vi "Sequence.vi"() -> ()   [LabVIEW 2016]
uses:
  Sequence.Action.ctl
  Sequence.Data.ctl
  Sequence.State.ctl
  Sequence.Step.Status.ctl
  Sequence.Test.BreakReason.ctl
  Sequence.Test.BreakSource.ctl
  Sequence.Test.Status.ctl
  Sequence.Slot.StatusData.ctl
  Sequence.Test.Unload.Status.ctl
  Sequence.Prod.StatusData.ctl
  Sequence.UserActions.ctl
  Sequence.UserData.ctl
  Sequence.MainMode.ctl
  Gui/MainGui.TestOptions.ctl
  Sequence.Code.Sets.ctl
  Sequence.PlateType.ctl
  Logger/Logger.Variant.Sets.ctl
  Station/Station.Changeover.State.vi
  Station/Station.Plate.Properties.ctl
  Sequence.Code.SerialFormat.ctl
  Drivers/V7310/LowLevel/V7310.Job.Sets.ctl
  Sequence.Counters.ctl
  tools/CitTemplate/citTemplate.errData.ctl
  tools/EventLog/EventLog.EventSource.ctl
  tools/Translator/Translator.Message.ctl
  Station/Station.ValvePosition.ctl
  Drivers/FestoCPX/Station/FestoCPX.Station.ProdArmPosition.ctl
  Station/Station.ProductSlot.ctl
  Sequence.SerialsFglb.Action.ctl
  Sequence.UserAction.ctl
  Sequence.Global.vi
  Station/Station.Global.vi
  Drivers/V7310/LowLevel/V7310.Global.vi
panel:
  out "SuckerLastStates":bool[](array[boolean])
  out "Data":T1={"BeginTS"=timestamp(0 s since 1904-01-01), "EndTS"=timestamp(0 s since 1904-01-01), "State"=enum."Init", "Status.Work"=enum."-", "Status.Process"=enum."-", "Status.Home"=enum."-", "Status.Wabco"=enum."-", "Status.Client"=enum."-", "BreakReason"=enum."-", "BreakSource"=enum."-", "DoorLock"=FALSE, "Status.Prod"=[], "UserAction"={"Stop"=FALSE, "Pause"=FALSE, "Next"=FALSE}, "UserData"={"GuiMode"=enum."Process", "Test"={"IgnoreResults"=FALSE, "IgnoreImages"=FALSE, "ServiceMode"=FALSE}, "ContinueOrder"=FALSE}, "Error"={"status"=FALSE, "code"=0, "source"=""}, "Code"={"Ready"=FALSE, "DoubleOrder"=FALSE, "OrderDone"=FALSE, "AllowSingleSlot"=FALSE, "CheckDM"=FALSE, "ThresholdA"=0, "ThresholdB"=0, "Plate"=enum."Wabco", "ImgPath"=path "", "Variant"={"State"=enum."Init", "ImgPath"=path "", "WabcoPlate"="", "WabcoProduct"="", "ClientProduct"="", "ClientPlate"="", "TotalQuantity"=0, "OrderQuantity"=0, "Serial"=0, "Wabco"={"LaserJob"="", "AdditionalTxt"="037", "FactoryCode"="", "RevID"=0, "ForkID"=0, "FailuresLimit"=0, "GlobalCnt"=0, "ScannerProgram"=0, "SerialFormat"=enum."6 dig", "CoordA"={"X"=0.0, "Y"=0.0, "Angle"=0.0}, "CoordB"={"X"=0.0, "Y"=0.0, "Angle"=0.0}, "DMCconfig"=0}, "Client"={"LaserJob"="", "AdditionalTxt"="", "FactoryCode"="037", "RevID"=0, "ForkID"=0, "FailuresLimit"=0, "GlobalCnt"=0, "ScannerProgram"=0, "SerialFormat"=enum."6 dig", "CoordA"={"X"=0.0, "Y"=0.0, "Angle"=0.0}, "CoordB"={"X"=0.0, "Y"=0.0, "Angle"=0.0}, "DMCconfig"=0}}}, "Rotations"=0, "ProdIdx"=0, "ProdDone"=[], "PrintedSerials-Wabco"=[], "PrintedSerials-Client"=[], "Counters-Wabco"={"Expected"=0, "Done"=0, "OK"=0, "NOK"=0, "NOKlimit"=0, "Part"=0, "PartOK"=0}, "Counters-Client"={"Expected"=0, "Done"=0, "OK"=0, "NOK"=0, "NOKlimit"=0, "Part"=0, "PartOK"=0}}
  out "action":T22=enum."--- Sequence ---"
  out "_loop":i32(ring)=4
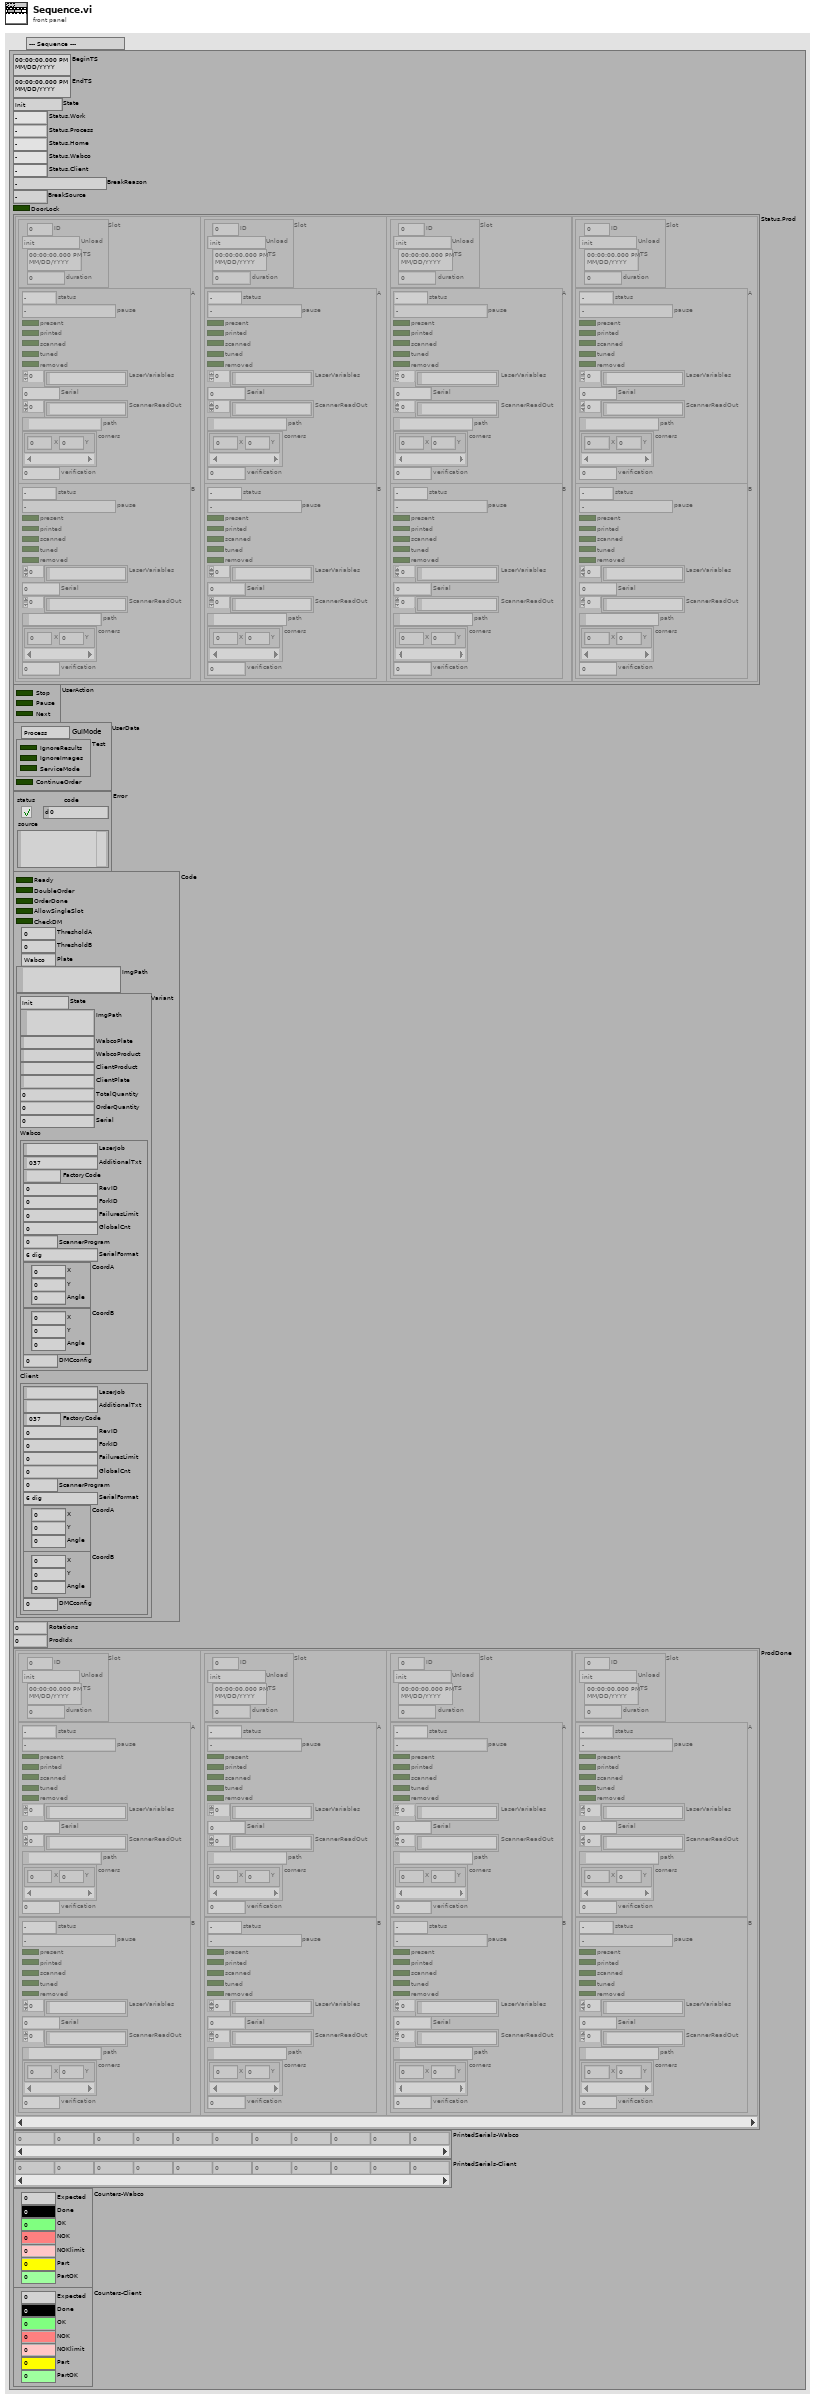
[diagram p1: front panel]
types:
  T1 = typedef "Sequence.Data.ctl" = cluster{"BeginTS":timestamp, "EndTS":timestamp, "State":T2, "Status.Work":T3, "Status.Process":T3, "Status.Home":T3, "Status.Wabco":T3, "Status.Client":T3, "BreakReason":T4, "BreakSource":T5, "DoorLock":bool, "Status.Prod":T6[], "UserAction":T10, "UserData":T11, "Error":errorcluster, "Code":T14, "Rotations":i32, "ProdIdx":i32, "ProdDone":T6[], "PrintedSerials-Wabco":i32[], "PrintedSerials-Client":i32[], "Counters-Wabco":T21, "Counters-Client":T21}
  T2 = typedef "Sequence.State.ctl" = enum16{"Init", "Idle", "Home", "Work", "Run", "Pause"}
  T3 = typedef "Sequence.Step.Status.ctl" = enum16{"-", "Pending", "Running", "Skipped", "Passed", "Failed", "Done", "Error", "Aborted", "Stopped"}
  T4 = typedef "Sequence.Test.BreakReason.ctl" = enum16{"-", "NOK container", "OK container", "Rev empty", "Rev missing", "Rev wrong", "Fork missing", "Fork wrong", "NOK limit", "Unload failure", "Single slot", "Part done", "Err: Prod move work", "Err: Prod move home", "Err: Prod lift work", "Err: Prod lift home", "Err: Prod Arm Work", "Err: Prod Arm NOK", "Err: Prod Arm OK", "Err: Prod NOK suck", "Err: Prod NOK drop", "Err: Prod OK missing", "Err: Prod OK suck", "Err: Prod OK drop"}
  T5 = typedef "Sequence.Test.BreakSource.ctl" = enum16{"-", "A", "B", "A/B"}
  T6 = typedef "Sequence.Test.Status.ctl" = cluster{"Slot":T7, "A":T9, "B":T9}
  T7 = typedef "Sequence.Slot.StatusData.ctl" = cluster{"ID":i32, "Unload":T8, "TS":timestamp, "duration":u32}
  T8 = typedef "Sequence.Test.Unload.Status.ctl" = enum16{"init", "check NOK", "check OK", "wait on NOK", "wait on OK", "wait on Unload", "done"}
  T9 = typedef "Sequence.Prod.StatusData.ctl" = cluster{"status":T3, "pause":T4, "present":bool, "printed":bool, "scanned":bool, "tuned":bool, "removed":bool, "LaserVariables":string[], "Serial":i32, "ScannerReadOut":string[], "path":path, "corners":cluster{"X":i32, "Y":i32}[], "verification":u8}
  T10 = typedef "Sequence.UserActions.ctl" = cluster{"Stop":bool, "Pause":bool, "Next":bool}
  T11 = typedef "Sequence.UserData.ctl" = cluster{"GuiMode":T12, "Test":T13, "ContinueOrder":bool}
  T12 = typedef "Sequence.MainMode.ctl" = enum16{"Process", "Base", "Order", "Manual", "Logs", "Results", "Stats", "DMC Config"}
  T13 = typedef "MainGui.TestOptions.ctl" = cluster{"IgnoreResults":bool, "IgnoreImages":bool, "ServiceMode":bool}
  T14 = typedef "Sequence.Code.Sets.ctl" = cluster{"Ready":bool, "DoubleOrder":bool, "OrderDone":bool, "AllowSingleSlot":bool, "CheckDM":bool, "ThresholdA":u8, "ThresholdB":u8, "Plate":T15, "ImgPath":path, "Variant":T16}
  T15 = typedef "Sequence.PlateType.ctl" = enum16{"Wabco", "Client"}
  T16 = typedef "Logger.Variant.Sets.ctl" = cluster{"State":T17, "ImgPath":path, "WabcoPlate":string, "WabcoProduct":string, "ClientProduct":string, "ClientPlate":string, "TotalQuantity":u16, "OrderQuantity":u16, "Serial":i32, "Wabco":T18, "Client":T18}
  T17 = typedef "Station.Changeover.State.vi" = enum16{"Init", "Scaning", "NOK", "Wait for ack", "Ready"}
  T18 = typedef "Station.Plate.Properties.ctl" = cluster{"LaserJob":string, "AdditionalTxt":string, "FactoryCode":string, "RevID":u8, "ForkID":u8, "FailuresLimit":u16, "GlobalCnt":i32, "ScannerProgram":u8, "SerialFormat":T19, "CoordA":T20, "CoordB":T20, "DMCconfig":i32}
  T19 = typedef "Sequence.Code.SerialFormat.ctl" = enum8{"", "6 dig", "7 dig"}
  T20 = typedef "V7310.Job.Sets.ctl" = cluster{"X":dbl, "Y":dbl, "Angle":dbl}
  T21 = typedef "Sequence.Counters.ctl" = cluster{"Expected":u16, "Done":u16, "OK":u16, "NOK":u16, "NOKlimit":u16, "Part":u16, "PartOK":u16}
  T22 = typedef "Sequence.Action.ctl" = enum32{"idle", "constructor", "destructor", "--- Sequence ---", "Abort", "Init", "Select", "Start", "Work.Run", "Work.AirON", "Work.LaserON", "Work.Done", "Process.Run", "Process.Engine", "Process.Pause", "Process.DoorLock", "Process.Wait4Container", "Process.Wait1", "Process.Wait2", "Process.Continue", "Process.Done", "Home.Run", "Home.AirON", "Home.TablePos", "Home.MoveServo", "Home.LaserOFF", "Home.AirOFF", "Home.Done", "User.Action", "User.Data", "Status.Clear"}
  T23 = typedef "citTemplate.errData.ctl" = cluster{"ts":timestamp, "src":T24, "instance":i32, "action":string, "error":errorcluster, "unconfirmed":bool}
  T24 = typedef "EventLog.EventSource.ctl" = enum16{"All", "Gui", "Ref", "File", "Arch", "Seq", "CPX", "DB", "Laser", "Scan.P", "Scan.O"}
  T25 = typedef "Translator.Message.ctl" = enum16{"-", "Event confirmed", "Log out", "Log in", "Shutdown", "Cancel", "Start", "Begin time", "End time", "Duration", "Service Mode", "Ignore Results", "Serial Format", "On", "Off", "OK", "NOK", "NOK %s", "Home", "Work", "Close", "Open", "In progress...", "Missing", "Empty", "Hardware failure", "Initial", "Default", "Total", "Out of range", "Free disk space is below 1GB - contact technician", "Error %d >> %s", "Error %d >> %s >> %s", "Msg %d >> %s", "Laser msg %d %s", "Laser cmd error %s %d", "Laser cmd failed %s", "Laser cmd warning %s", "Laser disconnected", "Laser status %s", "Laser already started", "Laser job unkonwn %s", "Laser job missing %s", "Laser job select failure %s", "Unable to start laser printing (%s)", "Unable to stop laser printing (%s)", "Laser marking aborted", "Laser marking timeout", "Unable to reset Laser Interlock (%s)", "Unable to trigger Laser. Laser not ready (%s)", "Laser job '%s' coordinates not configured", "Starting %s", "Quitting %s", "Configured", "Initializing", "Quitting", "Loading", "Loaded %d results", "Loaded %d events", "Running", "Stopped", "Summary", "Laser", "Do you want to continue?", "Do you want to delete the configuration?", "The configuration is being used by an order. Unable to delete!", "Press confirm button", "Station is not based. Do you want to exit?", "Station requires changeover. Do you want to run the test?", "Test options are not set as default. Do you want to continue?", "Formatting of WabcoNo is disabled. Do you want to continue?", "Product not detected. Do you want to continue?", "Product scan failed. Do you want to continue?", "Calibration", "Log out?", "System", "All", "IDLE", "Translating...%s", "Not found", "Alarm %s", "Run", "Skip", "Abort", "Repeat", "Please wait...", "Database disconnected", "Database disconnected - changeover disabled!", "Login to database successful", "Login to database failed: %d; %s", "Unable to check the product status of reference %d - database disconnected", "Unable to set the product status of reference %d - database disconnected", "Variant file backup %s", "Read variant (%s)", "Result", "Station armed!", "Station requires changeover!", "Select reference number...", "EMERGENCY BUTTON - press Control button", "EMERGENCY DOOR - press Control button", "Resetting Emergency...", "Unable to reset safety circuit - Emergency Button pressed", "Unable to reset safety circuit - Emergency Side Door open", "Station not based", "Station based", "Station not empty", "Station basing...", "No order", "Press Start to begin new order", "Scanning new order", "Order NOK. Correct or scan again", "Order OK. Press Accept", "Order ready", "Revolver incorrect", "Fork incorrect", "Revolver missing", "Revolver empty", "Container missing", "Offline results", "Offline statistics", "Updating statistics %.1f %%", "DMC Configurator", "Door open", "Close the front door", "Press start button", "Done. Open the front door", "Running...", "Running...%.1f %%", "Pause %s", "Pause %s. NOK container missing", "Pause %s. OK container missing", "Pause %s. Revolver empty", "Pause %s. Revolver missing", "Pause %s. Revolver incorrect", "Pause %s. Fork missing", "Pause %s. Fork incorrect", "Pause %s. Too many failures", "Pause %s. Unloading failure", "Pause %s. One slot is not working", "Pause %s. Part order is done. Empty OK container", "Pause %s. Unable to move product to slot", "Pause %s. Unable to move back product pusher", "Pause %s. Unable to lift product", "Pause %s. Unable to move back product lifter", "Pause %s. Unable to move product arm to Work", "Pause %s. Unable to move product arm to NOK", "Pause %s. Unable to move product arm to OK", "Pause %s. Unable to unsuck the NOK product", "Pause %s. Unable to drop the NOK product", "Pause %s. Product OK missing", "Pause %s. Unable to unsuck the OK product", "Pause %s. Unable to drop the OK product", "Stopping...", "File '%s' is missing", "File '%s' is broken", "File '%s' is running", "Log file started (%s)", "Log file ended (%s)", "Log file stopped (%s)", "Log file ignored (%s)", "Log file exported (%s)", "Log file export failed (%s)", "Wrong serial number in log file", "Wrong reference number in log file", "Test steps are missing", "%s = %.3f", "Process param '%s' not found in DB", "Process param '%s' wrong order", "Process param '%s' value %.3f out of limits (%.3f; %.3f)", "Step%d param '%s' not found in DB", "Step%d param '%s' wrong order", "Step%d param '%s' value %.3f out of limits (%.3f; %.3f)", "Step%d EV '%s' not found in DB", "Step%d EV '%s' wrong order", "\"%s\" not found in DB", "\"%s\" wrong order", "\"%s\" value %.3f out of limits (%.3f; %.3f)", "\"%s\" not found in software", "Process init (%s)", "Process started", "Process restarted", "Process run", "Process done", "Process done - remove OK container", "Process aborted", "Process aborted at work", "Process aborted at home", "Process error", "Process error at home", "Process error at work", "Process close", "Process pause", "Process continue", "Process door open", "Process door close", "Process pause at slot %s due to %s", "Select plate from the order to process", "Do you want to start the process?", "Do you want to continue the process?", "There is unfinished order. Do you want to put the new order?", "Product %s %d OK", "Product %s %d NOK", "Unable to unload the slot %s. Product missing in the slot", "Unable to unload the slot %s. Product already in the arm", "Unable to accept the product as OK. Product missing in slot %s", "Unable to accept the product as OK. Product could not drop into the container at slot %s", "Unable to accept the product as NOK. Product could not drop into the container at slot %s", "Scan failed. Error %s", "Scan failed. Scanner disconnected", "Scan failed. Wrong Wabco number %d, limit (%d,%d)", "Scan failed. Wrong serial number %d, limit (%d,%d)", "Scan failed. Wrong date %d, limit (%d,%d)", "Scan failed. Wrong product wabco number %d (expected %d)", "Scan failed. Wrong product serial number %d (expected > 0)", "Scan OK %s", "Scan failed. Unable to determine table position (%s)", "Scan failed. Timeout", "Tune failed. Scanner disconnected", "Tune failed. Timeout", "%s = %d", "%s = %d->%d", "Unable to set %s = %.2f - Air Pressure Inside off", "Unable to set digital output '%s' = %d", "Unable to activate air pressure inside - timeout", "Unable to activate air pressure inside - aborted", "Unable to switch on Air Main Valve - Air Pressure Inlet off", "Unable to switch on Air Main Valve - Door open", "Unable to switch off Air Main Valve - timeout", "Unable to switch off Air Main Valve - aborted", "Unable to rotate Table - timeout", "Unable to rotate Table - aborted", "Unable to rotate Table - Product Move not in Home position", "Unable to rotate Table - Air Pressure Inside off", "Unable to rotate Table - Product Lift A not in Home position", "Unable to rotate Table - Product Lift B not in Home position", "Unable to rotate Table - unlock before movement timeout", "Unable to rotate Table - lock after movement timeout", "Unable to move Table Lock to %s position - timeout", "Unable to move Table Lock to %s position - aborted", "Unable to move Table Lock to %s position - Air Pressure Inside off", "Unable to move Table Lock to %s position - Table not in position", "Unable to move Product Lift A to %s position - timeout", "Unable to move Product Lift B to %s position - timeout", "Unable to move Product Lift A to %s position - aborted", "Unable to move Product Lift B to %s position - aborted", "Unable to move Product Lift A to %s position - Air Pressure Inside off", "Unable to move Product Lift B to %s position - Air Pressure Inside off", "Unable to move Product Lift A to %s position - Table not locked", "Unable to move Product Lift B to %s position - Table not locked", "Unable to move Product Lift A to %s position - Product Arm not in Work position", "Unable to move Product Lift B to %s position - Product Arm not in Work position", "Unable to set Product Suction Gripper %s to %s - timeout", "Unable to set Product Suction Gripper %s to %s - aborted", "Unable to set Product Suction Gripper %s to %s - Air Pressure Inside off", "Unable to set Product Suction Gripper %s to %s - Table slot unkown", "Unable to move Product Arm to %s position - timeout", "Unable to move Product Arm to %s position - aborted", "Unable to move Product Arm to %s position - Air Pressure Inside off", "Unable to move Product Arm to %s position - Product Lift A not in Home position", "Unable to move Product Arm to %s position - Product Lift B not in Home position", "Unable to move Product to %s position - timeout", "Unable to move Product to %s position - aborted", "Unable to move Product to %s position - Air Pressure Inside off", "Unable to move Product to %s position - Table not in position"}
  T26 = typedef "Station.ValvePosition.ctl" = enum16{"Home", "Work"}
  T27 = typedef "Station.ProductSlot.ctl" = enum8{"A", "B"}
  T28 = typedef "FestoCPX.Station.ProdArmPosition.ctl" = enum16{"Work", "OK", "NOK"}
  T29 = typedef "Sequence.SerialsFglb.Action.ctl" = enum16{"init", "get", "get next", "pass", "fail", "confirm", "clean"}
  T30 = typedef "Sequence.UserAction.ctl" = enum16{"-", "Stop", "Pause", "Continue", "Next"}
  T31 = typedef "citTemplate.notifierHandle.ctl" = refnum<notifier>
  T32 = typedef "FestoCPX.Station.ProdPresent.ctl" = cluster{"Slot1":cluster{"A":bool, "B":bool}, "Slot2":cluster{"A":bool, "B":bool}, "Slot3":cluster{"A":bool, "B":bool}, "Slot4":cluster{"A":bool, "B":bool}, "Final":cluster{"A":bool, "B":bool}, "OK":cluster{"A":bool, "B":bool}, "Container":cluster{"OK":bool, "NOK":bool}}
  T33 = typedef "Station.Buttons.ctl" = cluster{"Start":bool, "Stop":bool, "Control":bool}
  T34 = typedef "FestoCPX.Station.EmgState.ctl" = cluster{"Button":bool, "SideDoor":bool, "FrontDoor":bool, "DoorSecured":bool}
  T35 = typedef "V7310.Data.Status.ctl" = cluster{"State":T36, "LaserStatus":T37, "LaserStatusRaw":string, "Ref":refnum<k5>, "RTC TS":timestamp, "Conn TS":timestamp, "Msg":T38[], "JobInUse":string, "Jobs":string[], "Vars":T39[]}
  T36 = typedef "V7310.Data.Status.State.ctl" = enum16{"First", "Init", "Msg", "Error", "Abort", "Idle", "Run"}
  T37 = typedef "V7310.LaserStatus.ctl" = enum16{"-", "FatalError", "Initialize", "KeySwitchOpen", "TimeoutInterlock", "InterlockOpen", "StartUp", "ShutterlockOpen", "Standby", "Ready", "PrepareForMarking", "WaitForTrigger", "Marking"}
  T38 = typedef "V7310.Message.Data.ctl" = cluster{"ID":i32, "Msg":string}
  T39 = typedef "V7310.Job.Variable.ctl" = cluster{"Name":string, "Value":string}
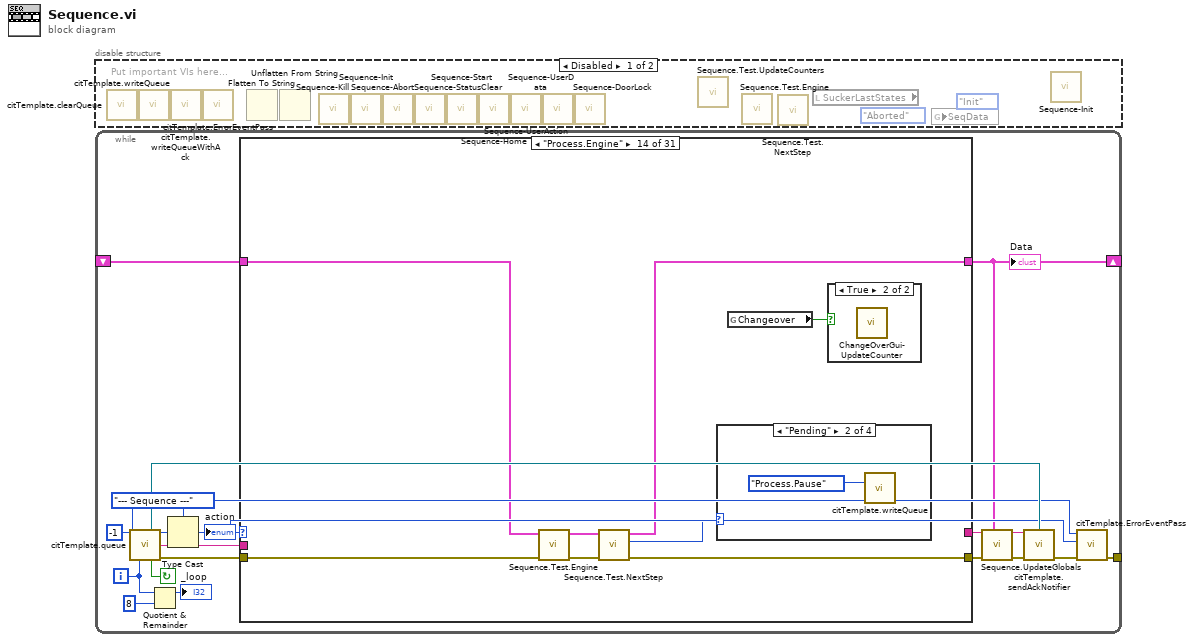
[diagram p0: block diagram]
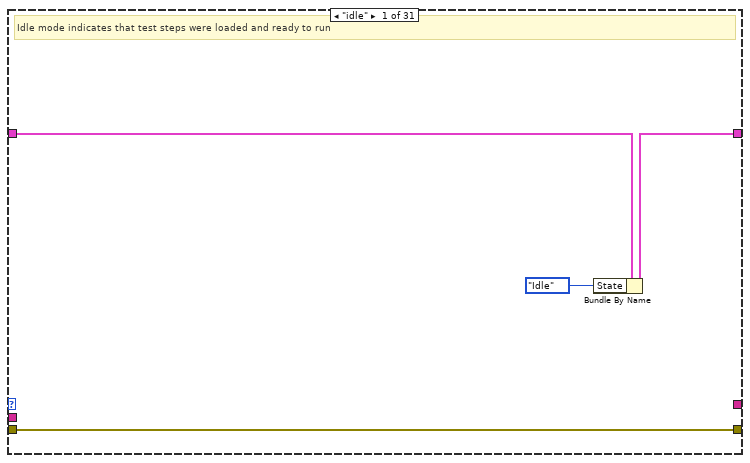
[diagram p3: hidden frame]
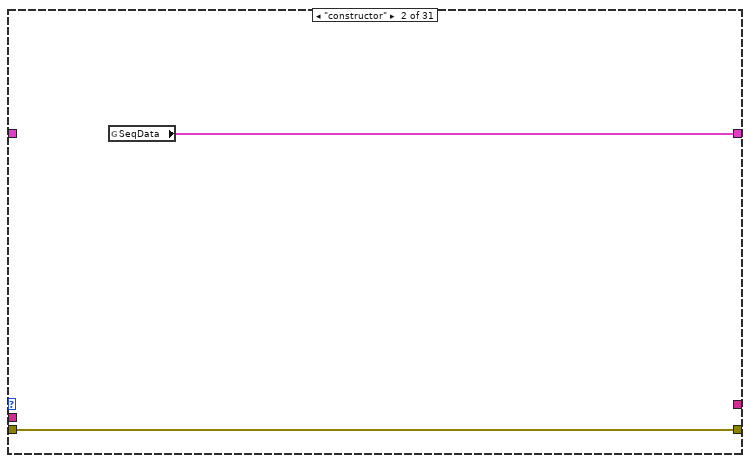
[diagram p4: hidden frame]
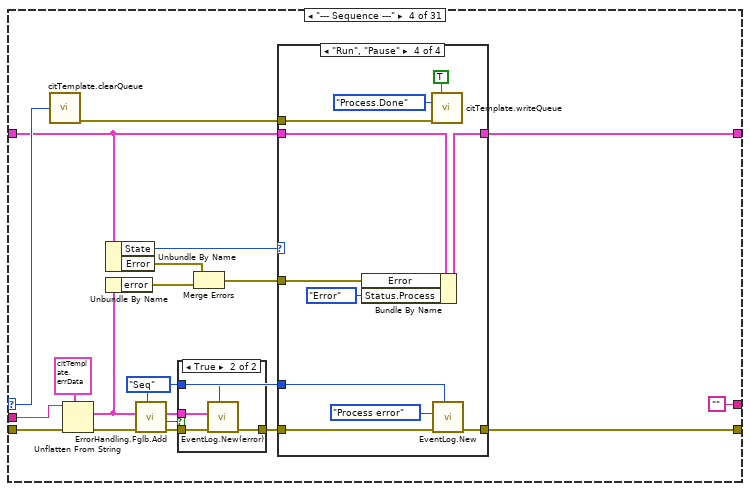
[diagram p6: hidden frame]
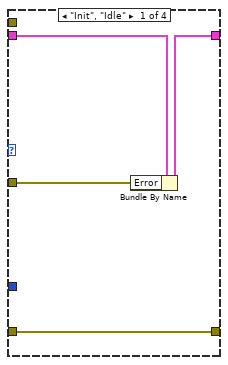
[diagram p7: hidden frame]
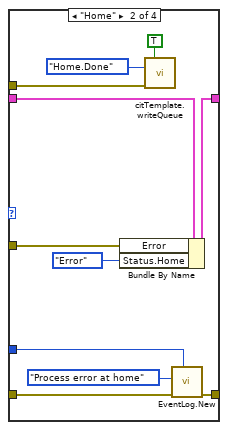
[diagram p8: hidden frame]
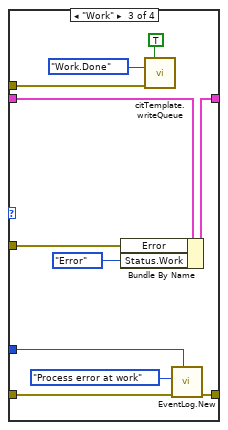
[diagram p9: hidden frame]
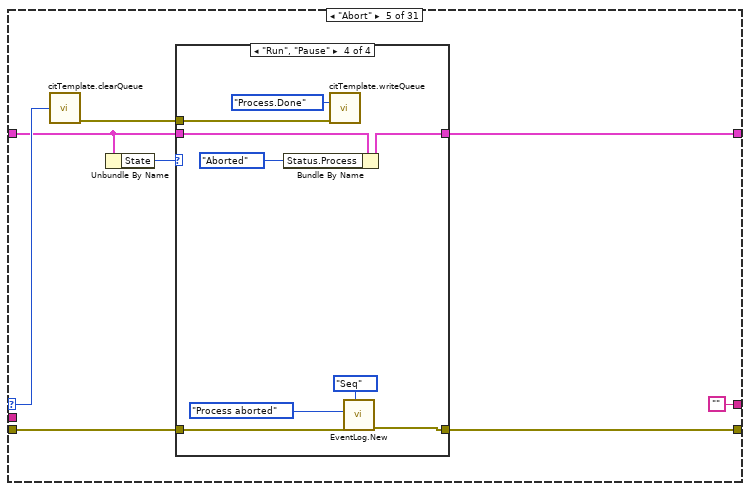
[diagram p11: hidden frame]
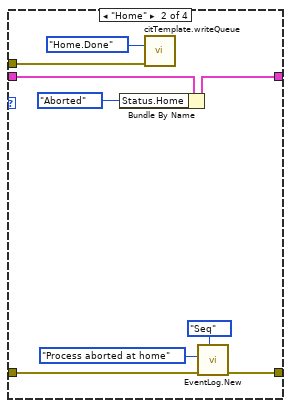
[diagram p13: hidden frame]
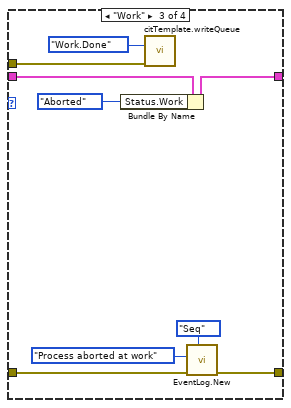
[diagram p14: hidden frame]
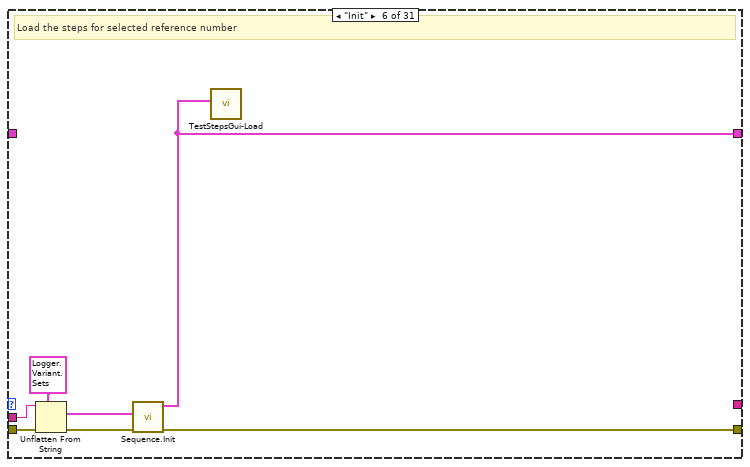
[diagram p15: hidden frame]
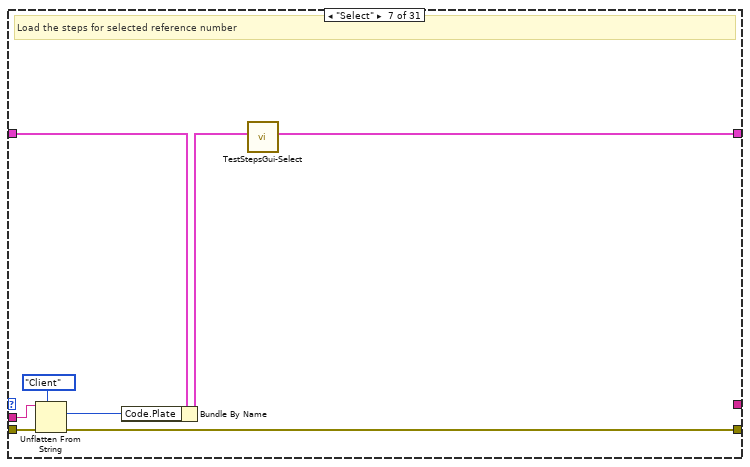
[diagram p16: hidden frame]
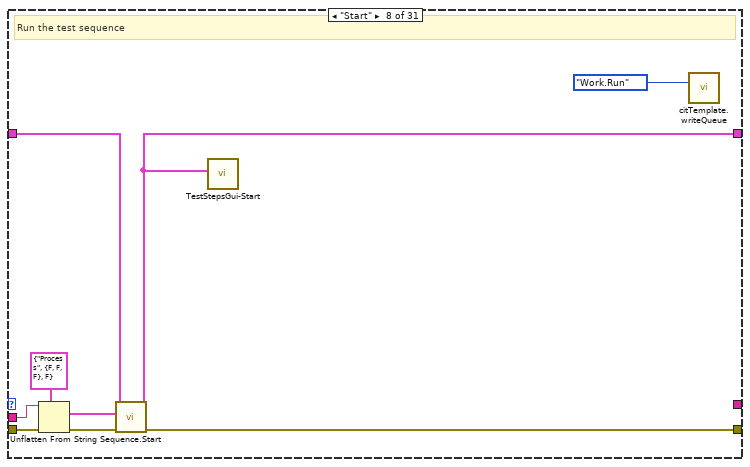
[diagram p17: hidden frame]
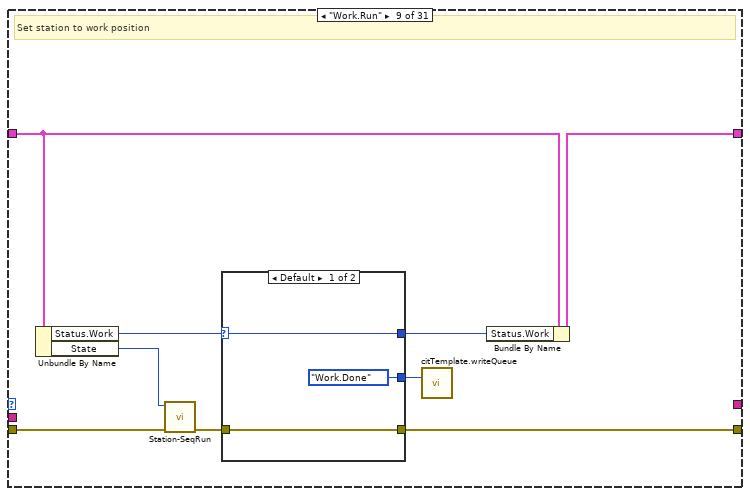
[diagram p18: hidden frame]
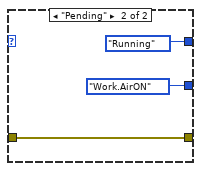
[diagram p19: hidden frame]
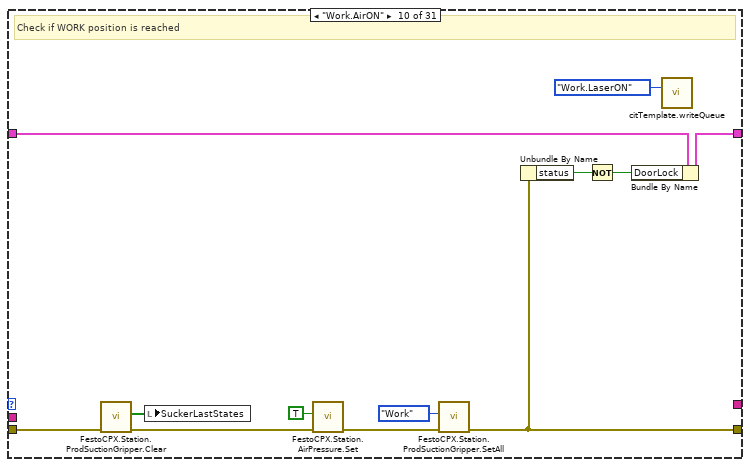
[diagram p20: hidden frame]
diagram:
  n1 = disable-structure shown="Disabled" {
    frame Disabled {
      (unwired) Sequence.Step.Status."Aborted" ("Status")
      (unwired) Sequence.State."Init" ("State")
      # "Put important VIs here..."
      n2 = call "citTemplate.clearQueue.vi"() -> ()  [unwired: 14 in, 2 out]
      n3 = call "citTemplate.writeQueue.vi"() -> ()  [unwired: 15 in, 1 out]
      n4 = call "citTemplate.writeQueueWithAck.vi"() -> ()  [unwired: 13 in, 3 out]
      n5 = call "citTemplate.ErrorEventPass.vi"() -> ()  [unwired: 11 in, 1 out]
      n6 = Flatten To String() -> ()  [unwired: 4 in, 3 out]
      n7 = Unflatten From String() -> ()  [unwired: 5 in, 3 out]
      n8 = call "Sequence-Kill.vi"() -> ()  [unwired: 11 in, 1 out]
      n9 = call "Sequence-Init.vi"() -> ()  [unwired: 11 in, 1 out]
      n10 = call "Sequence-Abort.vi"() -> ()  [unwired: 11 in, 1 out]
      n11 = call "Sequence-StatusClear.vi"() -> ()  [unwired: 11 in, 1 out]
      n12 = call "Sequence-Start.vi"() -> ()  [unwired: 11 in, 1 out]
      n13 = call "Sequence-Home.vi"() -> ()  [unwired: 11 in, 1 out]
      n14 = call "Sequence-UserAction.vi"() -> ()  [unwired: 11 in, 1 out]
      n15 = call "Sequence-UserData.vi"() -> ()  [unwired: 11 in, 1 out]
      n16 = call "Sequence-DoorLock.vi"() -> ()  [unwired: 11 in, 1 out]
      n17 = call "Sequence.Test.UpdateCounters.vi"() -> ()  [unwired: 9 in, 3 out]
      n18 = call "Sequence.Test.Engine.vi"() -> ()  [unwired: 10 in, 2 out]
      n19 = call "Sequence.Test.NextStep.vi"() -> ()  [unwired: 9 in, 3 out]
      n20 = local read "SuckerLastStates"() -> ()  [unwired: 1 out]
      n21 = global read "Sequence.Global.vi" "SeqData"() -> ()  [unwired: 1 in]
      n22 = call "Sequence-Init.vi"() -> ()  [unwired: 11 in, 1 out]
    }
    frame Enabled {
    }
  }
  n23 = while {
    tunnel: [w6] -> _
    shift-right: [w2] -> _
    shift-left: _ -> [w4]
    i -> [w8]
    stop <- w14 continue-if-true
    w11 = Sequence.Action."--- Sequence ---" ("Action")
    n24 = call "citTemplate.queue.vi"("ms timeout (250 ms)"=-1, "event enum"=w11, "iteration (-1)"=w8) -> ("notifierHandle out"=w13:T31, "event out"=w17:u32, "(flatten) data out"=w16:string, "continue"=w14:bool, "error out"=w15:errorcluster)  [unwired: 2 in, 6 out]
    n25 = Quotient & Remainder(x=w8, y=8) -> (x-y*floor(x/y)=→"_loop":i32)  [unwired: 1 out]
    n26 = Type Cast(type=w11, x=w17) -> (*(type *) &x=w7:T22)
    "action" <- w7
    n27 = case shown="\"Process.Engine\"" w7 {
      selector: w7 -> [_ _ _ w35 w93 _ _ _ _ _ _ _ _ _ _ _ _ _ _ _ _ _ _ _ _ _ _ _ _ _ _]
      tunnel: w16 -> [_ _ _ w43 _ w129 w136 w144 _ _ _ _ _ _ _ w245 _ _ _ _ _ _ _ _ _ _ _ _ w499 w528 _]
      tunnel: w15 -> [w18 w23 w24 w42 w87 w130 w137 w145 w149 w169 w178 w185 w197 w210 w224 w250 w284 w309 w336 w350 w391 w392 w399 w420 w434 w462 w473 w484 w501 w529 w530]
      tunnel: [_ _ _ "" "" _ _ _ _ _ _ _ _ _ _ _ _ _ _ _ _ _ _ _ _ _ _ _ _ _ _] -> w12
      tunnel: [w18 w23 w24 w26 w90 w127 w132 w143 w150 w164 w175 w186 w201 w207 w223 w249 w280 w307 w334 w347 w387 w392 w398 w426 w448 w464 w476 w483 w500 w523 w530] -> w3
      tunnel: [w21 w22 w25 w31 w88 w128 w131 w141 w155 w165 w177 w184 w200 w208 w229 w247 w285 w294 w317 w363 w386 w395 w401 w425 w447 w468 w469 w482 w502 w527 w531] -> w2
      tunnel: w4 -> [w20 _ w25 w32 w89 _ w134 w138 w154 w166 w177 w187 w199 w205 w228 w248 w286 w295 w318 w360 w390 w396 w402 w425 w447 w468 w471 w485 w497 w524 w532]
      frame "idle" {
        # "Idle mode indicates that test steps were loaded and ready to run"
        n28 = Bundle By Name(cluster=w20, "State"=Sequence.State."Idle") -> (w21:T1)
      }
      frame "constructor" {
        n29 = global read "Sequence.Global.vi" "SeqData"() -> (w22:T1)
      }
      frame "destructor" {
      }
      frame "--- Sequence ---" {
        w27 = EventLog.EventSource."Seq" ("Event source")
        n30 = call "citTemplate.clearQueue.vi"("event in"=w35) -> ("error out"=w34:errorcluster)  [unwired: 13 in, 1 out]
        n31 = Unflatten From String(type=T23 {"ts"=timestamp(0 s since 1904-01-01), "src"=enum."All", "instance"=0, "action"="", "error"={"status"=FALSE, "code"=0, "source"=""}, "unconfirmed"=FALSE} ("ErrData"), binary string=w43, error in (no error)=w42) -> (value=w37:T23, error out=w38:errorcluster)  [unwired: 3 out]
        n32 = Unbundle By Name(w32) -> ("State"=w33:T2, "Error"=w30:errorcluster)
        n33 = Unbundle By Name(w37) -> ("error"=w36:errorcluster)
        n34 = call "ErrorHandling.Fglb.Add.vi"("Event source"=w27, "error in (no error)"=w38, "Error in"=w37) -> ("error out"=w40:errorcluster, "changed?"=w39:bool)  [unwired: 7 in]
        n35 = case shown="True" w39 {
          tunnel: [w82 w86] -> w28
          tunnel: w37 -> [_ w85]
          tunnel: w40 -> [w82 w84]
          tunnel: w27 -> [_ w83]
          frame False {
          }
          frame True {
            n36 = call "EventLog.New(error).vi"("Source (All)"=w83, "error in"=w84, "ErrData"=w85) -> ("error out"=w86:errorcluster)  [unwired: 8 in]
          }
        }
        n37 = Merge Errors(w30, w36) -> (w29:errorcluster)
        n38 = case shown="\"Run\", \"Pause\"" w33 {
          tunnel: w34 -> [_ w57 w68 w80]
          tunnel: w28 -> [w48 w56 w67 w75]
          tunnel: [w48 w55 w66 w74] -> w26
          tunnel: w32 -> [w47 w53 w64 w79]
          tunnel: [w45 w52 w63 w78] -> w31
          tunnel: w29 -> [w46 w51 w62 w77]
          tunnel: w27 -> [_ w50 w61 w72]
          frame "Init", "Idle" {
            n39 = Bundle By Name(cluster=w47, "Error"=w46) -> (w45:T1)
          }
          frame "Home" {
            n40 = Bundle By Name(cluster=w53, "Error"=w51, "Status.Home"=Sequence.Step.Status."Error" ("Status")) -> (w52:T1)
            n41 = call "citTemplate.writeQueue.vi"("High priority (F)"=TRUE, "event in (if not connected:all statemachine with data event)"=Sequence.Action."Home.Done" ("Action"), "error in (no error)"=w57) -> ()  [unwired: 12 in, 1 out]
            n42 = call-poly "EventLog.New.vi"("Source (All)"=w50, "error in (no error)"=w56, "Message (-)"=Translator.Message."Process error at home" ("msg")) -> ("error out"=w55:errorcluster)  [unwired: 7 in, 1 out]
          }
          frame "Work" {
            n43 = Bundle By Name(cluster=w64, "Error"=w62, "Status.Work"=Sequence.Step.Status."Error" ("Status")) -> (w63:T1)
            n44 = call "citTemplate.writeQueue.vi"("High priority (F)"=TRUE, "event in (if not connected:all statemachine with data event)"=Sequence.Action."Work.Done" ("Action"), "error in (no error)"=w68) -> ()  [unwired: 12 in, 1 out]
            n45 = call-poly "EventLog.New.vi"("Source (All)"=w61, "error in (no error)"=w67, "Message (-)"=Translator.Message."Process error at work" ("msg")) -> ("error out"=w66:errorcluster)  [unwired: 7 in, 1 out]
          }
          frame "Run", "Pause" {
            n46 = Bundle By Name(cluster=w79, "Error"=w77, "Status.Process"=Sequence.Step.Status."Error" ("Status.Run")) -> (w78:T1)
            n47 = call "citTemplate.writeQueue.vi"("High priority (F)"=TRUE, "event in (if not connected:all statemachine with data event)"=Sequence.Action."Process.Done" ("Action"), "error in (no error)"=w80) -> ()  [unwired: 12 in, 1 out]
            n48 = call-poly "EventLog.New.vi"("Source (All)"=w72, "error in (no error)"=w75, "Message (-)"=Translator.Message."Process error" ("msg")) -> ("error out"=w74:errorcluster)  [unwired: 7 in, 1 out]
          }
        }
      }
      frame "Abort" {
        n49 = call "citTemplate.clearQueue.vi"("event in"=w93) -> ("error out"=w92:errorcluster)  [unwired: 13 in, 1 out]
        n50 = Unbundle By Name(w89) -> ("State"=w91:T2)
        n51 = case shown="\"Run\", \"Pause\"" w91 {
          tunnel: w92 -> [_ w103 w112 w122]
          tunnel: w87 -> [w96 w101 w110 w117]
          tunnel: [w96 w100 w109 w116] -> w90
          tunnel: w89 -> [w95 w98 w107 w121]
          tunnel: [w95 w97 w106 w120] -> w88
          frame "Init", "Idle" {
          }
          frame "Home" {
            n52 = Bundle By Name(cluster=w98, "Status.Home"=Sequence.Step.Status."Aborted" ("Status")) -> (w97:T1)
            n53 = call "citTemplate.writeQueue.vi"("event in (if not connected:all statemachine with data event)"=Sequence.Action."Home.Done" ("Action"), "error in (no error)"=w103) -> ()  [unwired: 13 in, 1 out]
            n54 = call-poly "EventLog.New.vi"("Source (All)"=EventLog.EventSource."Seq", "error in (no error)"=w101, "Message (-)"=Translator.Message."Process aborted at home" ("msg")) -> ("error out"=w100:errorcluster)  [unwired: 7 in, 1 out]
          }
          frame "Work" {
            n55 = Bundle By Name(cluster=w107, "Status.Work"=Sequence.Step.Status."Aborted" ("Status")) -> (w106:T1)
            n56 = call "citTemplate.writeQueue.vi"("event in (if not connected:all statemachine with data event)"=Sequence.Action."Work.Done" ("Action"), "error in (no error)"=w112) -> ()  [unwired: 13 in, 1 out]
            n57 = call-poly "EventLog.New.vi"("Source (All)"=EventLog.EventSource."Seq", "error in (no error)"=w110, "Message (-)"=Translator.Message."Process aborted at work" ("msg")) -> ("error out"=w109:errorcluster)  [unwired: 7 in, 1 out]
          }
          frame "Run", "Pause" {
            n58 = Bundle By Name(cluster=w121, "Status.Process"=Sequence.Step.Status."Aborted" ("Status.Run")) -> (w120:T1)
            n59 = call "citTemplate.writeQueue.vi"("event in (if not connected:all statemachine with data event)"=Sequence.Action."Process.Done" ("Action"), "error in (no error)"=w122) -> ()  [unwired: 13 in, 1 out]
            n60 = call-poly "EventLog.New.vi"("Source (All)"=EventLog.EventSource."Seq", "error in (no error)"=w117, "Message (-)"=Translator.Message."Process aborted" ("msg")) -> ("error out"=w116:errorcluster)  [unwired: 7 in, 1 out]
          }
        }
      }
      frame "Init" {
        # "Load the steps for selected reference number"
        n61 = Unflatten From String(type=T16 {"State"=enum."Init", "ImgPath"=path "", "WabcoPlate"="", "WabcoProduct"="", "ClientProduct"="", "ClientPlate"="", "TotalQuantity"=0, "OrderQuantity"=0, "Serial"=0, "Wabco"={"LaserJob"="", "AdditionalTxt"="037", "FactoryCode"="", "RevID"=0, "ForkID"=0, "FailuresLimit"=0, "GlobalCnt"=0, "ScannerProgram"=0, "SerialFormat"=enum."6 dig", "CoordA"={"X"=0.0, "Y"=0.0, "Angle"=0.0}, "CoordB"={"X"=0.0, "Y"=0.0, "Angle"=0.0}, "DMCconfig"=0}, "Client"={"LaserJob"="", "AdditionalTxt"="", "FactoryCode"="037", "RevID"=0, "ForkID"=0, "FailuresLimit"=0, "GlobalCnt"=0, "ScannerProgram"=0, "SerialFormat"=enum."6 dig", "CoordA"={"X"=0.0, "Y"=0.0, "Angle"=0.0}, "CoordB"={"X"=0.0, "Y"=0.0, "Angle"=0.0}, "DMCconfig"=0}} ("VariantSets"), binary string=w129, error in (no error)=w130) -> (value=w124:T16, error out=w126:errorcluster)  [unwired: 2 in, 1 out]
        n62 = call "Sequence.Init.vi"("error in (no error)"=w126, "VariantSets"=w124) -> ("error out"=w127:errorcluster, "Data out"=w128:T1)  [unwired: 8 in]
        n63 = call "TestStepsGui-Load.vi"("Data"=w128) -> ()  [unwired: 10 in, 1 out]
      }
      frame "Select" {
        # "Load the steps for selected reference number"
        n64 = Unflatten From String(type=Sequence.PlateType."Client" ("PlateType"), binary string=w136, error in (no error)=w137) -> (value=w133:T15, error out=w132:errorcluster)  [unwired: 2 in, 1 out]
        n65 = Bundle By Name(cluster=w134, "Code.Plate"=w133) -> (w131:T1)
        n66 = call "TestStepsGui-Select.vi"("Data"=w131) -> ()  [unwired: 10 in, 1 out]
      }
      frame "Start" {
        # "Run the test sequence"
        n67 = Unflatten From String(type=T11 {"GuiMode"=enum."Process", "Test"={"IgnoreResults"=FALSE, "IgnoreImages"=FALSE, "ServiceMode"=FALSE}, "ContinueOrder"=FALSE} ("SeqOptions"), binary string=w144, error in (no error)=w145) -> (value=w139:T11, error out=w142:errorcluster)  [unwired: 2 in, 1 out]
        n68 = call "Sequence.Start.vi"("error in"=w142, "UserSets"=w139, "Data in"=w138) -> ("error out"=w143:errorcluster, "Data out"=w141:T1)  [unwired: 7 in]
        n69 = call "TestStepsGui-Start.vi"("Data"=w141) -> ()  [unwired: 10 in, 1 out]
        n70 = call "citTemplate.writeQueue.vi"("event in (if not connected:all statemachine with data event)"=Sequence.Action."Work.Run" ("Action")) -> ()  [unwired: 14 in, 1 out]
      }
      frame "Work.Run" {
        # "Set station to work position"
        n71 = Unbundle By Name(w154) -> ("Status.Work"=w153:T3, "State"=w147:T2)
        n72 = call "Station-SeqRun.vi"("error in (no error)"=w149, "State"=w147) -> ("error out"=w148:errorcluster)  [unwired: 9 in]
        n73 = case shown="Default" w153 {
          selector: w153 -> [w156 _]
          tunnel: w148 -> [w158 w159]
          tunnel: [w158 w159] -> w150
          tunnel: [w156 Sequence.Step.Status."Running" ("Status")] -> w152
          tunnel: [Sequence.Action."Work.Done" ("Action") Sequence.Action."Work.AirON" ("Action")] -> w151
          frame Default {
          }
          frame "Pending" {
          }
        }
        n74 = call "citTemplate.writeQueue.vi"("event in (if not connected:all statemachine with data event)"=w151) -> ()  [unwired: 14 in, 1 out]
        n75 = Bundle By Name(cluster=w154, "Status.Work"=w152) -> (w155:T1)
      }
      frame "Work.AirON" {
        # "Check if WORK position is reached"
        n76 = call "FestoCPX.Station.ProdSuctionGripper.Clear.vi"("error in"=w169) -> ("error out"=w168:errorcluster, "States before clear"=w167:bool[])  [unwired: 9 in]
        n77 = local write "SuckerLastStates"(w167) -> ()
        n78 = call "FestoCPX.Station.AirPressure.Set.vi"("error in"=w168, "State"=TRUE ("Lock")) -> ("error out"=w170:errorcluster)  [unwired: 9 in]
        n79 = call "FestoCPX.Station.ProdSuctionGripper.SetAll.vi"("error in"=w170, "Position"=Station.ValvePosition."Work") -> ("error out"=w164:errorcluster)  [unwired: 9 in]
        n80 = Unbundle By Name(w164) -> ("status"=w163:bool)
        n81 = Not(x=w163) -> (.not. x?=w162:bool)
        n82 = Bundle By Name(cluster=w166, "DoorLock"=w162) -> (w165:T1)
        n83 = call "citTemplate.writeQueue.vi"("event in (if not connected:all statemachine with data event)"=Sequence.Action."Work.LaserON" ("Action")) -> ()  [unwired: 14 in, 1 out]
      }
      frame "Work.LaserON" {
        w174 = TRUE ("Interlock")
        n84 = call "FestoCPX.Station.Laser.Interlock.vi"("error in"=w178, "Wait (T)"=w174, "Interlock"=w174) -> ("error out"=w176:errorcluster)  [unwired: 8 in]
        n85 = call "FestoCPX.Station.Laser.FumeExtractUnit.vi"("error in"=w176, "FumeExtractUnit"=w174) -> ("error out"=w175:errorcluster)  [unwired: 9 in]
        n86 = call "citTemplate.writeQueue.vi"("event in (if not connected:all statemachine with data event)"=Sequence.Action."Work.Done" ("Action")) -> ()  [unwired: 14 in, 1 out]
      }
      frame "Work.Done" {
        # "Machine in WORK position - Execute Test Sequence"
        n87 = Unbundle By Name(w187) -> ("Status.Process"=w183:T3, "Status.Work"=w189:T3)
        n88 = case shown="\"Skipped\", \"Error\"..\"Stopped\"" w189 {
          selector: w189 -> [_ w194]
          tunnel: [Sequence.Action."Process.Run" ("Action") Sequence.Action."Process.Done" ("Action")] -> w188
          tunnel: [Sequence.Step.Status."Done" ("Work.Status") w194] -> w180
          tunnel: w183 -> [_ w193]
          tunnel: [Sequence.Step.Status."Pending" ("Status.Test") w193] -> w182
          frame Default {
          }
          frame "Skipped", "Error".."Stopped" {
          }
        }
        n89 = Bundle By Name(cluster=w187, "Status.Process"=w182, "Status.Work"=w180) -> (w184:T1)
        n90 = call "citTemplate.writeQueue.vi"("event in (if not connected:all statemachine with data event)"=w188) -> ()  [unwired: 14 in, 1 out]
        n91 = call "Station-SeqDone.vi"("error in (no error)"=w185, "Status"=w180, "State"=Sequence.State."Work") -> ("error out"=w186:errorcluster)  [unwired: 8 in]
      }
      frame "Process.Run" {
        n92 = Unbundle By Name(w199) -> ("State"=w198:T2)
        n93 = call "Station-SeqRun.vi"("error in (no error)"=w197, "State"=w198) -> ("error out"=w196:errorcluster)  [unwired: 9 in]
        n94 = call "Sequence.Test.Init.vi"("error in"=w196, "Data in"=w199) -> ("error out"=w201:errorcluster, "Data out"=w200:T1)  [unwired: 8 in]
        n95 = call "citTemplate.writeQueue.vi"("event in (if not connected:all statemachine with data event)"=Sequence.Action."Process.Engine" ("Action")) -> ()  [unwired: 14 in, 1 out]
      }
      frame "Process.Engine" {
        n96 = call "Sequence.Test.Engine.vi"("error in (no error)"=w210, "Data in"=w205) -> ("error out"=w209:errorcluster, "Data out"=w206:T1)  [unwired: 8 in]
        n97 = call "Sequence.Test.NextStep.vi"("error in"=w209, "Data in"=w206) -> ("error out"=w207:errorcluster, "Final Status"=w204:T3, "Data out"=w208:T1)  [unwired: 7 in]
        n98 = case shown="\"Pending\"" w204 {
          frame Default {
            n99 = Wait (ms)(milliseconds to wait=u32 50) -> ()  [unwired: 1 out]
            n100 = call "citTemplate.writeQueue.vi"("event in (if not connected:all statemachine with data event)"=Sequence.Action."Process.Engine" ("Action")) -> ()  [unwired: 14 in, 1 out]
          }
          frame "Pending" {
            n101 = call "citTemplate.writeQueue.vi"("event in (if not connected:all statemachine with data event)"=Sequence.Action."Process.Pause" ("Action")) -> ()  [unwired: 14 in, 1 out]
          }
          frame "Done" {
            n102 = call "citTemplate.writeQueue.vi"("event in (if not connected:all statemachine with data event)"=Sequence.Action."Process.Done" ("Action")) -> ()  [unwired: 14 in, 1 out]
          }
          frame "Error".."Stopped" {
            n103 = call "citTemplate.writeQueue.vi"("event in (if not connected:all statemachine with data event)"=Sequence.Action."Process.Done" ("Action")) -> ()  [unwired: 14 in, 1 out]
          }
        }
        n104 = global read "Station.Global.vi" "Changeover"() -> (w203:bool)
        n105 = case shown="True" w203 {
          frame False {
          }
          frame True {
            n106 = call "ChangeOverGui-UpdateCounter.vi"() -> ()  [unwired: 11 in, 1 out]
          }
        }
      }
      frame "Process.Pause" {
        n107 = Unbundle By Name(w228) -> ("BreakReason"=w217:T4, "BreakSource"=w222:T5)
        n108 = Format Into String(w217) -> (resulting string=w220:string)  [unwired: 3 in, 1 out]
        n109 = Format Into String(w222) -> (resulting string=w221:string)  [unwired: 3 in, 1 out]
        n110 = To Variant(anything=w221) -> (Variant=w219:variant)
        n111 = To Variant(anything=w220) -> (Variant=w216:variant)
        n112 = Equal?(x=w217, y=Sequence.Test.BreakReason."Part done") -> (x = y?=w226:bool)
        n113 = Build Array(w219, w216) -> (w218:variant[])
        n114 = case shown="True" w226 {
          tunnel: [Sequence.Action."Process.Wait1" ("Action") Sequence.Action."Process.Wait4Container" ("Action")] -> w225
          frame False {
          }
          frame True {
          }
        }
        n115 = case shown="Default" w217 {
          tunnel: w224 -> [w235 w237]
          tunnel: [w234 w236] -> w223
          tunnel: w218 -> [w233 _]
          frame Default {
            n116 = call "EventLog.New(array).vi"("Source (All)"=EventLog.EventSource."Seq", "error in (no error)"=w235, "Arguments"=w233, "Message (-)"=Translator.Message."Process pause at slot %s due to %s") -> ("error out"=w234:errorcluster)  [unwired: 6 in, 1 out]
          }
          frame "-" {
            n117 = call "EventLog.New(array).vi"("Source (All)"=EventLog.EventSource."Seq", "error in (no error)"=w237, "Message (-)"=Translator.Message."Process pause") -> ("error out"=w236:errorcluster)  [unwired: 7 in, 1 out]
          }
        }
        n118 = Bundle By Name(cluster=w228, "State"=Sequence.State."Pause") -> (w229:T1)
        n119 = call "citTemplate.writeQueue.vi"("event in (if not connected:all statemachine with data event)"=w225) -> ()  [unwired: 14 in, 1 out]
      }
      frame "Process.DoorLock" {
        n120 = Unflatten From String(type=FALSE, binary string=w245, error in (no error)=w250) -> (value=w243:bool, error out=w246:errorcluster)  [unwired: 2 in, 1 out]
        n121 = case shown="False" w243 {
          tunnel: [w267 w273] -> w249
          tunnel: w246 -> [w257 w272]
          tunnel: [_ w277] -> w242
          frame False {
            w260 = Station.ValvePosition."Home" ("Position")
            n122 = call "FestoCPX.Station.ProdLift.Move.vi"("error in"=w257, "Position"=w260, "Slot"=Station.ProductSlot."A") -> ("error out"=w259:errorcluster)  [unwired: 8 in]
            n123 = call "FestoCPX.Station.ProdLift.Move.vi"("error in"=w257, "Position"=w260, "Slot"=Station.ProductSlot."B") -> ("error out"=w258:errorcluster)  [unwired: 8 in]
            n124 = Merge Errors(w259, w258) -> (w256:errorcluster)
            n125 = call "FestoCPX.Station.ProdArm.Move.vi"("error in"=w256, "Product Status"=FestoCPX.Station.ProdArmPosition."Work") -> ("error out"=w254:errorcluster)  [unwired: 9 in]
            n126 = call "Wait (with error).vi"("error in (no error)"=w254, "milliseconds to wait"=u32 500) -> ("error out"=w253:errorcluster)  [unwired: 8 in, 1 out]
            n127 = call <vilib>:"Clear Errors.vi"("error in (no error)"=w253) -> ("error out"=w263:errorcluster)  [unwired: 5 in, 1 out]
            n128 = call "EventLog.New(array).vi"("Source (All)"=EventLog.EventSource."Seq", "Message (-)"=Translator.Message."Process door open") -> ()  [unwired: 8 in, 2 out]
            n129 = call "FestoCPX.Station.ProdSuctionGripper.Clear.vi"("error in"=w263) -> ("error out"=w265:errorcluster, "States before clear"=→"SuckerLastStates":bool[])  [unwired: 9 in]
            n130 = call "FestoCPX.Station.AirPressure.Set.vi"("error in"=w265, "State"=FALSE ("Lock")) -> ("error out"=w267:errorcluster)  [unwired: 9 in]
          }
          frame True {
            n131 = call "FestoCPX.Station.AirPressure.Set.vi"("error in"=w272, "State"=TRUE ("Lock")) -> ("error out"=w271:errorcluster)  [unwired: 9 in]
            n132 = local read "SuckerLastStates"() -> (w276:bool[])
            n133 = call "EventLog.New(array).vi"("Source (All)"=EventLog.EventSource."Seq", "Message (-)"=Translator.Message."Process door close") -> ()  [unwired: 8 in, 2 out]
            n134 = call "FestoCPX.Station.ProdSuctionGripper.Restore.vi"("error in"=w271, "States before clear"=w276) -> ("error out"=w273:errorcluster)  [unwired: 9 in]
            n135 = Unbundle By Name(w273) -> ("status"=w275:bool)
            n136 = Not(x=w275) -> (.not. x?=w277:bool)
          }
        }
        n137 = Bundle By Name(cluster=w248, "DoorLock"=w242) -> (w247:T1)
      }
      frame "Process.Wait4Container" {
        # "wait for door open to fix problem or start button to continue"
        n138 = call "FestoCPX.Station.ProdPresent.Check.vi"("error in"=w284) -> ("error out"=w280:errorcluster, "Prod Present"=w283:T32)  [unwired: 5 in, 4 out]
        n139 = Unbundle By Name(w286) -> ("UserAction.Stop"=w289:bool)
        n140 = Unbundle By Name(w283) -> ("Container.OK"=w279:bool)
        n141 = feedback-in #1(w279) -> ()
        n142 = feedback #1(w279) -> (w282:bool)
        n143 = Compound Arithmetic op=AND(w279, invert w282) -> (w278:bool)
        n144 = Wait (ms)(milliseconds to wait=u32 50) -> ()  [unwired: 1 out]
        n145 = Select(t=Sequence.Action."Process.Wait1" ("Action"), s=w278, f=Sequence.Action."Process.Wait4Container" ("Action")) -> (s? t:f=w281:T22)
        n146 = Select(t=Sequence.Action."Process.Engine" ("Action"), s=w289, f=w281) -> (s? t:f=w288:T22)
        n147 = call "citTemplate.writeQueue.vi"("event in (if not connected:all statemachine with data event)"=w288) -> ()  [unwired: 14 in, 1 out]
        n148 = Bundle By Name(cluster=w286, "State"=Sequence.State."Pause") -> (w285:T1)
      }
      frame "Process.Wait1" {
        # "wait for door open to fix problem or start button to continue"
        n149 = Unbundle By Name(w295) -> ("UserAction.Stop"=w300:bool, "State"=w305:T2)
        n150 = call "Station.Buttons.Check.vi"("error in"=w309) -> ("error out"=w308:errorcluster, "Buttons"=w310:T33)  [unwired: 8 in, 1 out]
        n151 = Unbundle By Name(w310) -> ("Start"=w315:bool)
        n152 = Equal?(x=w305, y=Sequence.State."Run") -> (x = y?=w302:bool)
        n153 = call "FestoCPX.Station.Emg.Check.vi"("error in"=w308) -> ("error out"=w307:errorcluster, "Emg"=w306:T34)  [unwired: 8 in, 1 out]
        n154 = Unbundle By Name(w306) -> ("FrontDoor"=w299:bool)
        n155 = Compound Arithmetic op=OR(w302, w315) -> (w303:bool)
        n156 = Wait (ms)(milliseconds to wait=u32 50) -> ()  [unwired: 1 out]
        n157 = Select(t=Sequence.Action."Process.Continue" ("Action"), s=w303, f=Sequence.Action."Process.Wait1" ("Action")) -> (s? t:f=w311:T22)
        n158 = Select(t=w311, s=w299, f=Sequence.Action."Process.Wait2" ("Action")) -> (s? t:f=w298:T22)
        n159 = Select(t=Sequence.Action."Process.Engine" ("Action"), s=w300, f=w298) -> (s? t:f=w297:T22)
        n160 = call "citTemplate.writeQueue.vi"("event in (if not connected:all statemachine with data event)"=w297) -> ()  [unwired: 14 in, 1 out]
        n161 = Bundle By Name(cluster=w295, "State"=Sequence.State."Pause") -> (w294:T1)
      }
      frame "Process.Wait2" {
        # "wait for door close and start button to continue"
        n162 = Unbundle By Name(w318) -> ("UserAction.Stop"=w322:bool, "State"=w328:T2)
        n163 = call "Station.Buttons.Check.vi"("error in"=w336) -> ("error out"=w335:errorcluster, "Buttons"=w337:T33)  [unwired: 8 in, 1 out]
        n164 = Unbundle By Name(w337) -> ("Start"=w332:bool)
        n165 = call "FestoCPX.Station.Emg.Check.vi"("error in"=w335) -> ("error out"=w334:errorcluster, "Emg"=w333:T34)  [unwired: 8 in, 1 out]
        n166 = Equal?(x=w328, y=Sequence.State."Run") -> (x = y?=w326:bool)
        n167 = Unbundle By Name(w333) -> ("FrontDoor"=w331:bool)
        n168 = Compound Arithmetic op=OR(w326, w332) -> (w329:bool)
        n169 = Wait (ms)(milliseconds to wait=u32 50) -> ()  [unwired: 1 out]
        n170 = Compound Arithmetic op=AND(w329, invert w331) -> (w325:bool)
        n171 = Select(t=Sequence.Action."Process.Continue" ("Action"), s=w325, f=Sequence.Action."Process.Wait2" ("Action")) -> (s? t:f=w323:T22)
        n172 = Select(t=Sequence.Action."Process.Engine" ("Action"), s=w322, f=w323) -> (s? t:f=w320:T22)
        n173 = call "citTemplate.writeQueue.vi"("event in (if not connected:all statemachine with data event)"=w320) -> ()  [unwired: 14 in, 1 out]
        n174 = Bundle By Name(cluster=w318, "State"=Sequence.State."Pause") -> (w317:T1)
      }
      frame "Process.Continue" {
        w343 = T4[] [enum."NOK limit", enum."Part done"] items=["-", "NOK container", "OK container", "Rev empty", "Rev missing", "Rev wrong", "Fork missing", "Fork wrong", "NOK limit", "Unload failure", "Single slot", "Part done", "Err: Prod move work", "Err: Prod move home", "Err: Prod lift work", "Err: Prod lift home", "Err: Prod Arm Work", "Err: Prod Arm NOK", "Err: Prod Arm OK", "Err: Prod NOK suck", "Err: Prod NOK drop", "Err: Prod OK missing", "Err: Prod OK suck", "Err: Prod OK drop"] ("appended array")
        w358 = Sequence.Test.BreakReason."Single slot" ("x")
        n175 = Unbundle By Name(w360) -> ("Code.AllowSingleSlot"=w355:bool, "Status.Prod"=w352:T6[], "DoorLock"=w351:bool)
        n176 = case shown="False" w351 {
          selector: w351 -> [_ w380]
          tunnel: [w375 w381] -> w348
          tunnel: w350 -> [w374 w381]
          tunnel: [w379 w380] -> w349
          frame False {
            n177 = call "FestoCPX.Station.AirPressure.Set.vi"("error in"=w374, "State"=TRUE ("Lock")) -> ("error out"=w373:errorcluster)  [unwired: 9 in]
            n178 = local read "SuckerLastStates"() -> (w378:bool[])
            n179 = call "FestoCPX.Station.ProdSuctionGripper.Restore.vi"("error in"=w373, "States before clear"=w378) -> ("error out"=w375:errorcluster)  [unwired: 9 in]
            n180 = Unbundle By Name(w375) -> ("status"=w377:bool)
            n181 = Not(x=w377) -> (.not. x?=w379:bool)
          }
          frame True {
          }
        }
        n182 = Index Array(array=w352) -> (element=w359:T6)  [unwired: 1 in]
        n183 = Unbundle By Name(w359) -> ("A.pause"=w346:T4, "B.pause"=w345:T4)
        n184 = Equal?(x=w358, y=w346) -> (x = y?=w357:bool)
        n185 = Build Array(w346, w345) -> (w344:T4[])
        n186 = Equal?(x=w358, y=w345) -> (x = y?=w356:bool)
        n187 = Compound Arithmetic op=OR(w357, w356) -> (w353:bool)
        n188 = for {
          tunnel: w344 -> [w368]
          tunnel: w343 -> [w367] mode=indexing
          tunnel: [w365] -> w342 mode=indexing
          n189 = Search 1D Array(1D array=w368, element=w367) -> (index of element=w366:i32)  [unwired: 1 in]
          n190 = Greater Or Equal To 0?(x=w366) -> (x >= 0?=w365:bool)
        }
        n191 = call "EventLog.New(array).vi"("Source (All)"=EventLog.EventSource."Seq", "Message (-)"=Translator.Message."Process continue") -> ()  [unwired: 8 in, 2 out]
        n192 = Select(t=w353, s=w353, f=w355) -> (s? t:f=w354:bool)
        n193 = Or Array Elements(Boolean array=w342) -> (logical OR=w341:bool)
        n194 = case shown="True" w341 {
          tunnel: w348 -> [w369 w371]
          tunnel: [w369 w370] -> w347
          frame False {
          }
          frame True {
            n195 = call "Sequence.SerialsFglb.vi"("Action (get)"=Sequence.SerialsFglb.Action."confirm" ("Action"), "error in"=w371) -> ("error out"=w370:errorcluster)  [unwired: 5 in, 4 out]
          }
        }
        n196 = Bundle By Name(cluster=w360, "Code.AllowSingleSlot"=w354, "State"=Sequence.State."Run", "UserAction.Pause"=FALSE, "DoorLock"=w349) -> (w363:T1)
        n197 = call "citTemplate.writeQueue.vi"("event in (if not connected:all statemachine with data event)"=Sequence.Action."Process.Engine" ("Action")) -> ()  [unwired: 14 in, 1 out]
      }
      frame "Process.Done" {
        # "Sequence is completed (all test steps are done); home procedure is not done yet; collect sequence status and complete the log file"
        n198 = call "Sequence.Test.Done.vi"("error in"=w391, "Data in"=w390) -> ("error out"=w389:errorcluster, "Order done"=w382:bool, "Data out"=w386:T1)  [unwired: 7 in]
        n199 = call "Logger-End.vi"("error in"=w389, "SeqData"=w386) -> ("error out"=w388:errorcluster)  [unwired: 9 in]
        n200 = Unbundle By Name(w386) -> ("Status.Process"=w383:T3)
        n201 = call "TestStepsGui-Select.vi"("Data"=w386) -> ()  [unwired: 10 in, 1 out]
        n202 = call "Station-SeqDone.vi"("error in (no error)"=w388, "Order done (F)"=w382, "Status"=w383, "State"=Sequence.State."Run") -> ("error out"=w387:errorcluster)  [unwired: 7 in]
        n203 = global read "Station.Global.vi" "Changeover"() -> (w385:bool)
        n204 = case shown="True" w385 {
          frame False {
          }
          frame True {
            n205 = call "ChangeOverGui-UpdateCounter.vi"() -> ()  [unwired: 11 in, 1 out]
          }
        }
      }
      frame "Home.Run" {
        # "Initialize home/base procedure (check if VI is runnable)"
        n206 = Bundle By Name(cluster=w396, "State"=Sequence.State."Home", "Status.Home"=Sequence.Step.Status."Running" ("Status")) -> (w395:T1)
        n207 = call "citTemplate.writeQueue.vi"("event in (if not connected:all statemachine with data event)"=Sequence.Action."Home.AirON" ("Action")) -> ()  [unwired: 14 in, 1 out]
      }
      frame "Home.AirON" {
        # "Check if WORK position is reached"
        n208 = call "FestoCPX.Station.Emg.Check.vi"("error in"=w399) -> ("error out"=w406:errorcluster, "Emg"=w405:T34)  [unwired: 8 in, 1 out]
        n209 = Unbundle By Name(w405) -> ("FrontDoor"=w404:bool)
        n210 = case shown="False" w404 {
          tunnel: [w407 w415] -> w398
          tunnel: w406 -> [w411 w416]
          tunnel: [Sequence.Action."Home.TablePos" ("Action") Sequence.Action."Home.LaserOFF" ("Action")] -> w403
          tunnel: [w408 _] -> w400
          frame False {
            n211 = call "FestoCPX.Station.ProdSuctionGripper.Clear.vi"("error in"=w411) -> ("error out"=w410:errorcluster, "States before clear"=w412:bool[])  [unwired: 9 in]
            n212 = local write "SuckerLastStates"(w412) -> ()
            n213 = call "FestoCPX.Station.AirPressure.Set.vi"("error in"=w410, "State"=TRUE ("Lock")) -> ("error out"=w407:errorcluster)  [unwired: 9 in]
            n214 = Unbundle By Name(w407) -> ("status"=w409:bool)
            n215 = Not(x=w409) -> (.not. x?=w408:bool)
          }
          frame True {
            n216 = global read "Station.Global.vi" "ScannerSlot"() -> (w418:i32)
            n217 = call "Keyence.Main-GetTablePosition.vi"("error in (no error)"=w416, "ScannerSlot in"=w418) -> ("error out"=w415:errorcluster, "ScannerSlot out"=w417:i32)  [unwired: 7 in, 1 out]
            n218 = global write "Station.Global.vi" "ScannerSlot"(w417) -> ()
          }
        }
        n219 = call "citTemplate.writeQueue.vi"("event in (if not connected:all statemachine with data event)"=w403) -> ()  [unwired: 14 in, 1 out]
        n220 = Bundle By Name(cluster=w402, "DoorLock"=w400) -> (w401:T1)
      }
      frame "Home.TablePos" {
        n221 = call "FestoCPX.Station.Table.Check.vi"("error in"=w420) -> ("error out"=w423:errorcluster, "Table Lock"=w421:bool, "Table Pos"=w422:bool)  [unwired: 8 in]
        n222 = Compound Arithmetic op=OR(w422, invert w421) -> (w427:bool)
        n223 = case shown="True" w427 {
          tunnel: w423 -> [w431 w433]
          tunnel: [w431 w432] -> w428
          frame False {
          }
          frame True {
            n224 = call "FestoCPX.Station.Table.Rotate.vi"("error in"=w433) -> ("error out"=w432:errorcluster)  [unwired: 10 in]
          }
        }
        n225 = global read "Station.Global.vi" "ScannerSlot"() -> (w430:i32)
        n226 = call "citTemplate.writeQueue.vi"("event in (if not connected:all statemachine with data event)"=Sequence.Action."Home.MoveServo" ("Action")) -> ()  [unwired: 14 in, 1 out]
        n227 = call "Keyence.Main-GetTablePosition.vi"("error in (no error)"=w428, "Force (F)"=w427, "ScannerSlot in"=w430) -> ("error out"=w426:errorcluster, "ScannerSlot out"=w429:i32)  [unwired: 6 in, 1 out]
        n228 = global write "Station.Global.vi" "ScannerSlot"(w429) -> ()
      }
      frame "Home.MoveServo" {
        w439 = Station.ValvePosition."Home" ("Position")
        n229 = global read "V7310.Global.vi" "Laser.Status"() -> (w438:T35)
        n230 = Unbundle By Name(w438) -> ("State"=w436:T36, "LaserStatus"=w437:T37)
        n231 = case shown="\"Init\", \"Idle\"" w436 {
          tunnel: w437 -> [_ w454]
          tunnel: w434 -> [w451 w453]
          tunnel: [w451 w452] -> w435
          frame Default {
          }
          frame "Init", "Idle" {
            n232 = case shown="\"TimeoutInterlock\"" w454 {
              tunnel: w453 -> [w455 w461]
              tunnel: [w455 w459] -> w452
              frame Default {
              }
              frame "TimeoutInterlock" {
                n233 = call "FestoCPX.Station.Laser.Interlock.vi"("error in"=w461, "Wait (T)"=FALSE, "Interlock"=TRUE) -> ("error out"=w460:errorcluster)  [unwired: 8 in]
                n234 = call "Wait (with error).vi"("error in (no error)"=w460, "milliseconds to wait"=u32 2000) -> ("error out"=w459:errorcluster)  [unwired: 8 in, 1 out]
              }
            }
          }
        }
        n235 = call "FestoCPX.Station.ProdLift.Move.vi"("error in"=w434, "Position"=w439, "Slot"=Station.ProductSlot."A") -> ("error out"=w444:errorcluster)  [unwired: 8 in]
        n236 = call "FestoCPX.Station.ProdLift.Move.vi"("error in"=w434, "Position"=w439, "Slot"=Station.ProductSlot."B") -> ("error out"=w445:errorcluster)  [unwired: 8 in]
        n237 = call "FestoCPX.Station.ProdMove.Move.vi"("error in"=w434, "Position"=w439) -> ("error out"=w441:errorcluster)  [unwired: 8 in, 1 out]
        n238 = Merge Errors(w444, w445) -> (w443:errorcluster)
        n239 = call "FestoCPX.Station.ProdArm.Move.vi"("error in"=w443, "Product Status"=FestoCPX.Station.ProdArmPosition."Work") -> ("error out"=w442:errorcluster)  [unwired: 9 in]
        n240 = Merge Errors(w435, w442, w441) -> (w448:errorcluster)
        n241 = call "citTemplate.writeQueue.vi"("event in (if not connected:all statemachine with data event)"=Sequence.Action."Home.LaserOFF" ("Action")) -> ()  [unwired: 14 in, 1 out]
      }
      frame "Home.LaserOFF" {
        w463 = FALSE ("Shutterlock")
        n242 = call "FestoCPX.Station.Laser.Trigger.vi"("error in"=w462, "Wait (T)"=w463, "Trigger"=w463) -> ("error out"=w466:errorcluster)  [unwired: 7 in, 1 out]
        n243 = call "FestoCPX.Station.Laser.FumeExtractUnit.vi"("error in"=w466, "FumeExtractUnit"=w463) -> ("error out"=w465:errorcluster)  [unwired: 9 in]
        n244 = call "FestoCPX.Station.Laser.Interlock.vi"("error in"=w465, "Wait (T)"=w463, "Interlock"=w463) -> ("error out"=w464:errorcluster)  [unwired: 8 in]
        n245 = call "citTemplate.writeQueue.vi"("event in (if not connected:all statemachine with data event)"=Sequence.Action."Home.AirOFF" ("Action")) -> ()  [unwired: 14 in, 1 out]
      }
      frame "Home.AirOFF" {
        # "Check if WORK position is reached"
        n246 = call "FestoCPX.Station.ProdSuctionGripper.SetAll.vi"("error in"=w473, "Position"=Station.ValvePosition."Home") -> ("error out"=w472:errorcluster)  [unwired: 9 in]
        n247 = call "FestoCPX.Station.AirPressure.Set.vi"("error in"=w472, "State"=FALSE ("Lock")) -> ("error out"=w476:errorcluster)  [unwired: 9 in]
        n248 = Bundle By Name(cluster=w471, "DoorLock"=FALSE) -> (w469:T1)
        n249 = call "citTemplate.writeQueue.vi"("event in (if not connected:all statemachine with data event)"=Sequence.Action."Home.Done" ("Action")) -> ()  [unwired: 14 in, 1 out]
      }
      frame "Home.Done" {
        # "Home/base procedure is done"
        n250 = Unbundle By Name(w485) -> ("Status.Home"=w481:T3)
        n251 = case shown="\"Error\"..\"Stopped\"" w481 {
          selector: w481 -> [w486 _]
          tunnel: [w486 Sequence.Step.Status."Done" ("Home.Status")] -> w478
          frame "Error".."Stopped" {
          }
          frame Default {
          }
        }
        n252 = Bundle By Name(cluster=w485, "State"=Sequence.State."Idle", "Status.Home"=w478) -> (w482:T1)
        n253 = call "Station-SeqDone.vi"("error in (no error)"=w484, "Status"=w478, "State"=Sequence.State."Home") -> ("error out"=w483:errorcluster)  [unwired: 8 in]
      }
      frame "User.Action" {
        # "User pressed STOP button - wait until currently running substep is done and then abort"
        n254 = Unbundle By Name(w497) -> ("State"=w495:T2, "UserAction.Stop"=w490:bool, "UserAction.Pause"=w492:bool, "UserAction.Next"=w489:bool)
        n255 = Unflatten From String(type=Sequence.UserAction."Pause" ("UserAction"), binary string=w499, error in (no error)=w501) -> (value=w496:T30, error out=w500:errorcluster)  [unwired: 2 in, 1 out]
        n256 = case shown="\"Stop\"" w496 {
          tunnel: w495 -> [w503 w507 _ _ _]
          tunnel: [w503 w507 Sequence.State."Pause" ("State") Sequence.State."Run" ("State") Sequence.State."Run" ("State")] -> w494
          tunnel: [w504 TRUE w512 w517 w522] -> w493
          tunnel: [w505 w509 TRUE ("Pause") FALSE ("Pause") w521] -> w491
          tunnel: w492 -> [w505 w509 _ _ w521]
          tunnel: w490 -> [w504 _ w512 w517 w522]
          tunnel: w489 -> [w506 w508 w511 w515 _]
          tunnel: [w506 w508 w511 w515 TRUE] -> w488
          frame "-" {
          }
          frame "Stop" {
          }
          frame "Pause" {
          }
          frame "Continue" {
          }
          frame "Next" {
          }
        }
        n257 = Bundle By Name(cluster=w497, "State"=w494, "UserAction.Stop"=w493, "UserAction.Pause"=w491, "UserAction.Next"=w488) -> (w502:T1)
      }
      frame "User.Data" {
        # "User changed mode (Auto or Step)"
        n258 = Unflatten From String(type=T11 {"GuiMode"=enum."Process", "Test"={"IgnoreResults"=FALSE, "IgnoreImages"=FALSE, "ServiceMode"=FALSE}, "ContinueOrder"=FALSE} ("SeqOptions"), binary string=w528, error in (no error)=w529) -> (value=w525:T11, error out=w523:errorcluster)  [unwired: 2 in, 1 out]
        n259 = Bundle By Name(cluster=w524, "UserData"=w525) -> (w527:T1)
      }
      frame "Status.Clear" {
        n260 = Bundle By Name(cluster=w532, "Error"=w530) -> (w531:T1)
      }
    }
    "Data" <- w2
    n261 = call "Sequence.UpdateGlobals.vi"("SeqData"=w2, "error in"=w3) -> ("error out"=w1:errorcluster)  [unwired: 9 in]
    n262 = call "citTemplate.sendAckNotifier.vi"("notification data"=w12, "notifierHandle in"=w13, "error in"=w1) -> ()  [unwired: 13 out]
    n263 = call "citTemplate.ErrorEventPass.vi"("error in"=w1, "action of error"=w7, "event in"=w11) -> ("error out"=w6:errorcluster)  [unwired: 2 in, 6 out]
  }
